vi "Ex5stripGlueNI.vi"() -> ()   [LabVIEW 2010]
panel:
  in  "Upper wavelength":dbl=799.0 format="%.2f"
  in  "Lower wavelength":dbl=239.0 format="%.2f"
  in  "Glue Resolution":dbl=0.1 format="%.2f"
  in  "Flip":bool
  in  "Reverse":bool=TRUE
  in  "Intensifier Mode":enum16{"Safe", "Shutter", "Gate"}(ring)
  in  "Intensifier Gain":u32=100
  out "Glue":cluster{"Array":dbl[], "Array F32":sgl[]}(graph)
  in  "Calibration ini":path
  in  "ROI 5 Y2":u32=240
  in  "ROI 5 Y1":u32=208
  in  "ROI 4 Y2":u32=192
  in  "ROI 4 Y1":u32=160
  in  "ROI 3 Y2":u32=144
  in  "ROI 3 Y1":u32=112
  in  "ROI 2 Y2":u32=96
  in  "ROI 2 Y1":u32=64
  in  "ROI 1 Y2":u32=48
  in  "ROI 1 Y1":u32=16
  in  "Temperature":dbl=-10.0 format="%.2f"
  in  "Exposure":dbl=0.1 min=0.0 step=0.001 format="%.3f"
  in  "stop":bool
  out "error out":errorcluster
  in  "error in (no error)":errorcluster
  # "Calibration ini file"
  # "Ex5StripGlueNI.vi : this example shows the data collection of a frame with 5 strips and associates those strips with calibration supplied by a calibration ini file (which should have 5 segments of calibration defined). the graph color, exposure, and temperature can be entered at start."
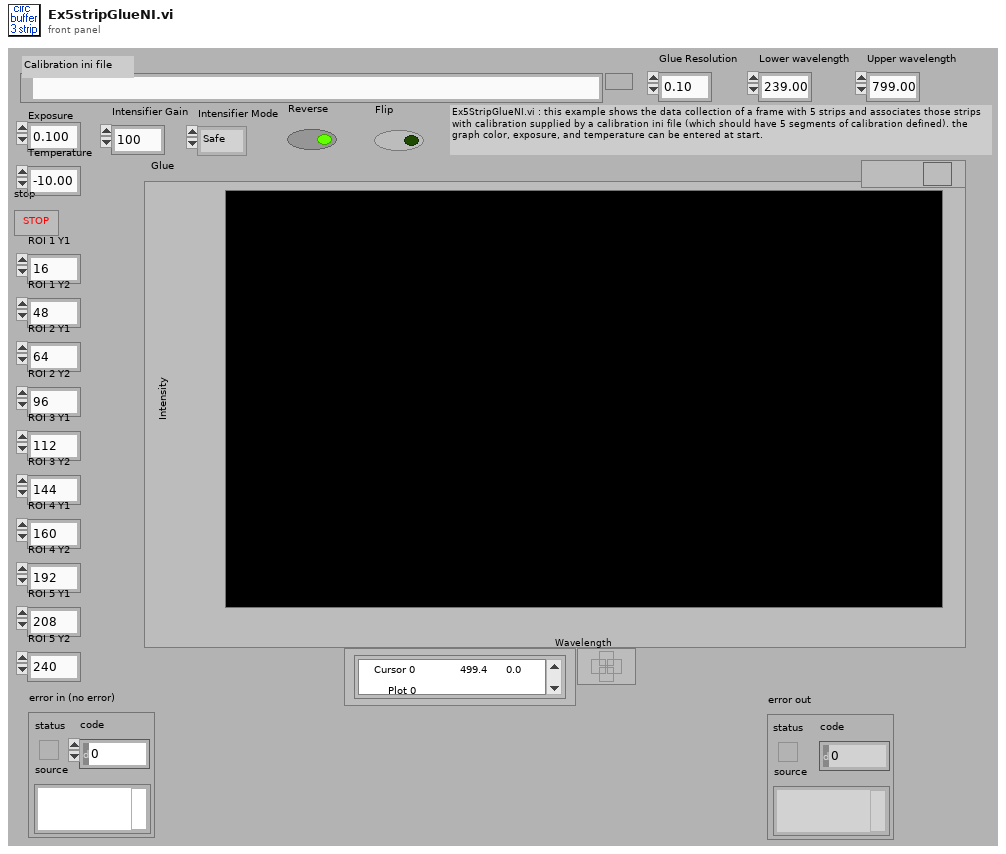
[diagram p1: front panel]
types:
  T1 = cluster{"ROI 1 Y1":u32, "ROI 1 Y2":u32, "ROI 2 Y1":u32, "ROI 2 Y2":u32, "ROI 3 Y1":u32, "ROI 3 Y2":u32, "ROI 4 Y1":u32, "ROI 4 Y2":u32, "ROI 5 Y1":u32, "ROI 5 Y2":u32}
  T2 = cluster{"Acquire focus mode,\nSync (circualar buffers)":i32, "Exposure":dbl, "Number of Images":i32, "Software Accumulation":i32}
  T3 = cluster{"Camera Handle":u32, "Pulser Handle":u32, "File Handle":u32, "Display Handle":u32, "Image Handle":u32}
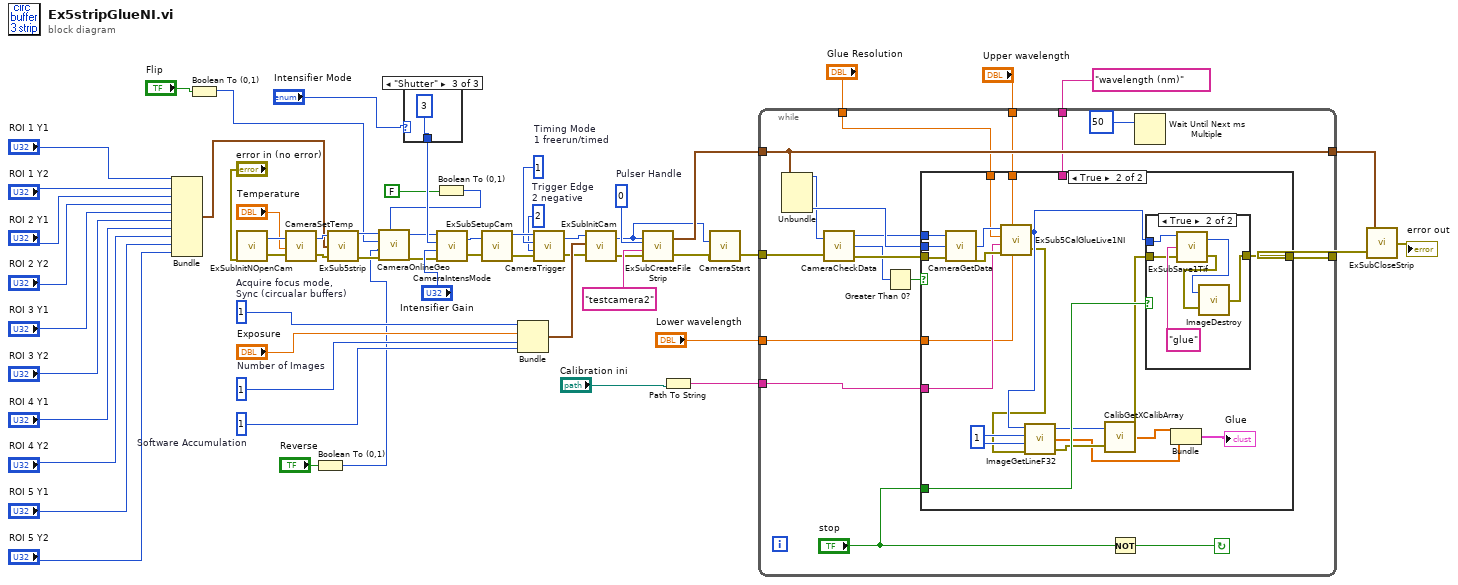
[diagram p0: block diagram]
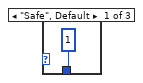
[diagram p2: hidden frame]
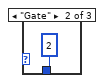
[diagram p3: hidden frame]
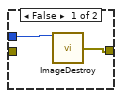
[diagram p5: hidden frame]
diagram:
  w42 = 2  # Trigger Edge 2 negative
  w43 = 1  # Timing Mode 1 freerun/timed
  w51 = 0  # Pulser Handle
  w57 = 1  # Number of Images
  w58 = 1  # Acquire focus mode, Sync (circualar buffers)
  w56 = 1  # Software Accumulation
  n1 = Bundle("ROI 1 Y1"="ROI 1 Y1", "ROI 1 Y2"="ROI 1 Y2", "ROI 2 Y1"="ROI 2 Y1", "ROI 2 Y2"="ROI 2 Y2", "ROI 3 Y1"="ROI 3 Y1", "ROI 3 Y2"="ROI 3 Y2", "ROI 4 Y1"="ROI 4 Y1", "ROI 4 Y2"="ROI 4 Y2", "ROI 5 Y1"="ROI 5 Y1", "ROI 5 Y2"="ROI 5 Y2") -> (w24:T1)  [unwired: 1 in]
  n2 = Boolean To (0,1)(Boolean="Flip") -> (0, 1=w6:i16)
  n3 = call "ExSubInitNOpenCam.vi"("error in (no error)"="error in (no error)") -> ("Camera Handle"=w37:u32, "error out"=w38:errorcluster)
  n4 = call <userlib>:"CameraSetTemp.vi"("error in (no error)"=w38, "Temperature"="Temperature", "Camera Handle"=w37) -> ("error out"=w39:errorcluster, "Camera Handle"=w36:u32)
  n5 = Boolean To (0,1)(Boolean="Reverse") -> (0, 1=w8:i16)
  n6 = call "ExSub5strip.vi"("error in (no error)"=w39, "5 ROIS"=w24, "Camera Handle"=w36) -> ("error out"=w12:errorcluster, "Camera Handle"=w11:u32)
  n7 = case shown="\"Shutter\"" "Intensifier Mode" {
    tunnel: [1 2 3] -> w14
    frame "Safe", Default {
    }
    frame "Gate" {
    }
    frame "Shutter" {
    }
  }
  n8 = Boolean To (0,1)(Boolean=FALSE) -> (0, 1=w5:i16)
  n9 = call <userlib>:"CameraOnlineGeo.vi"("Camera Handle"=w11, "Flip Flag"=w6, "Reverse Flag"=w8, "error in"=w12, "Rotate Flag"=w5) -> ("Camera Handle"=w10:u32, "error out"=w13:errorcluster)
  n10 = call <userlib>:"CameraIntensMode.vi"("error in"=w13, "Intensifier Gain"="Intensifier Gain", "Mode"=w14, "Camera Handle"=w10) -> ("error out"=w18:errorcluster, "Camera Handle"=w17:u32)
  n11 = call "ExSubSetupCam.vi"("error in (no error)"=w18, "Camera Handle"=w17) -> ("error out"=w41:errorcluster, "Camera Handle"=w45:u32)
  n12 = Bundle("Acquire focus mode,\nSync (circualar buffers)"=w58, "Exposure"="Exposure", "Number of Images"=w57, "Software Accumulation"=w56) -> (w53:T2)  [unwired: 1 in]
  n13 = call <userlib>:"CameraTrigger.vi"("error in"=w41, "Trigger Edge"=w42, "Timing Mode"=w43, "Camera Handle"=w45) -> ("error out"=w46:errorcluster, "Camera Handle"=w44:u32)
  n14 = call "ExSubInitCam.vi"("error in (no error)"=w46, "Camera Information"=w53, "Camera Handle"=w44) -> ("error out"=w52:errorcluster, "Camera Handle"=w49:u32)
  n15 = call "ExSubCreateFileStrip.vi"("error in (no error)"=w52, "File and Display Name"="testcamera2", "Pulser Handle"=w51, "Camera Handle"=w49) -> ("error out"=w19:errorcluster, "Handles Out"=w50:T3)
  n16 = Path To String(path="Calibration ini") -> (string=w22:string)
  n17 = call <userlib>:"CameraStart.vi"("error in"=w19, "Camera Handle"=w49) -> ("error out"=w40:errorcluster)  [unwired: 1 out]
  n18 = while {
    tunnel: w50 -> [w77]
    tunnel: w40 -> [w76]
    tunnel: [w74] -> w21
    tunnel: [w77] -> w48
    tunnel: w22 -> [w68]
    tunnel: "wavelength (nm)" -> [w66]
    tunnel: "Lower wavelength" -> [w65]
    tunnel: "Upper wavelength" -> [w64]
    tunnel: "Glue Resolution" -> [w63]
    stop <- w78 continue-if-true
    n19 = Unbundle(w77) -> ("Camera Handle"=w72:u32, "Image Handle"=w73:u32)  [unwired: 3 out]
    n20 = call <userlib>:"CameraCheckData.vi"("Camera Handle"=w72, "error in"=w76) -> ("Camera Handle"=w71:u32, "Number Of Frames Available"=w69:i32, "error out"=w75:errorcluster)
    n21 = Greater Than 0?(x=w69) -> (x > 0?=w70:bool)
    n22 = case shown="True" w70 {
      tunnel: w75 -> [w80 w100]
      tunnel: [w80 w94] -> w74
      tunnel: w73 -> [_ w99]
      tunnel: w71 -> [_ w98]
      tunnel: w68 -> [_ w93]
      tunnel: "stop" -> [_ w95]
      tunnel: w66 -> [_ _]
      tunnel: w65 -> [_ w83]
      tunnel: w64 -> [_ w82]
      tunnel: w63 -> [_ w81]
      frame False {
      }
      frame True {
        w91 = 1
        n23 = call <userlib>:"CameraGetData.vi"("error in"=w100, "Data Handle"=w99, "Camera Handle"=w98) -> ("error out"=w97:errorcluster, "Data Handle"=w96:u32)  [unwired: 1 out]
        n24 = call "ExSub5CalGlueLive1NI.vi"("Lower limit"=w83, "Upper limit"=w82, "error in (no error)"=w97, "String"=w93, "Resolution"=w81, "Image Handle"=w96) -> ("error out"=w90:errorcluster, "Glue handle"=w92:u32)
        n25 = call <userlib>:"ImageGetLineF32.vi"("error in"=w90, "Z Position"=w91, "Y Position"=w91, "Data Handle"=w92) -> ("error out"=w89:errorcluster, "Array F32"=w85:sgl[], "Data Handle"=w86:u32)
        n26 = call <userlib>:"CalibGetXCalibArray.vi"("Data Handle"=w86, "error in (no error)"=w89) -> ("Array"=w84:dbl[], "error out"=w88:errorcluster)  [unwired: 1 out]
        n27 = case shown="True" w95 {
          tunnel: w92 -> [w102 w108]
          tunnel: [w101 w104] -> w94
          tunnel: w88 -> [_ w103]
          frame False {
            n28 = call <userlib>:"ImageDestroy.vi"("Data handle"=w102) -> ("error out"=w101:errorcluster)  [unwired: 1 in]
          }
          frame True {
            n29 = call "ExSubSave1Tif.vi"("error in (no error)"=w103, "File name"="glue", "Image Handle"=w108) -> ("error out"=w106:errorcluster, "Image handle"=w105:u32)
            n30 = call <userlib>:"ImageDestroy.vi"("error in"=w106, "Data handle"=w105) -> ("error out"=w104:errorcluster)
          }
        }
        n31 = Bundle("Array"=w84, "Array F32"=w85) -> (→"Glue":cluster{"Array":dbl[], "Array F32":sgl[]})  [unwired: 1 in]
      }
    }
    n32 = Not(x="stop") -> (.not. x?=w78:bool)
    n33 = Wait Until Next ms Multiple(millisecond multiple=50) -> ()  [unwired: 1 out]
  }
  n34 = call "ExSubCloseStrip.vi"("error in (no error)"=w21, "Handles In"=w48) -> ("error out"=→"error out":errorcluster)
